vi "Ex 03 - A-Scan + Peaks (Live Update).vi"() -> ()   [LabVIEW 2015]
uses:
  <instrlib>/MicroPulse/Public/Data/Datatypes/MP - data formatting.ctl
  <instrlib>/MicroPulse/Public/Data/Datatypes/MP - amplitude reporting mode.ctl
  <instrlib>/MicroPulse/Public/Data/Datatypes/MP - averaging.ctl
  <instrlib>/MicroPulse/Public/Data/Datatypes/MP - transmit parameters.ctl
  <instrlib>/MicroPulse/Public/Data/Datatypes/MP - pulser voltage.ctl
  <instrlib>/MicroPulse/Public/Data/Datatypes/MP - pulse damping.ctl
  <instrlib>/MicroPulse/Public/Data/Datatypes/MP - test parameters.ctl
  <instrlib>/MicroPulse/Public/Data/Datatypes/MP - receive parameters.ctl
  <instrlib>/MicroPulse/Public/Data/Datatypes/MP - display gate.ctl
  <instrlib>/MicroPulse/Public/Data/Datatypes/MP - waveform type.ctl
  <instrlib>/MicroPulse/Public/Data/Datatypes/MP - analogue filter.ctl
  <instrlib>/MicroPulse/Public/Data/Datatypes/MP - frequency filter.ctl
  <instrlib>/MicroPulse/Public/Data/Datatypes/MP - digital filtering.ctl
  <instrlib>/MicroPulse/Public/Data/Datatypes/MP - high pass filter.ctl
  <instrlib>/MicroPulse/Public/Data/Datatypes/MP - low pass filter.ctl
  <instrlib>/MicroPulse/Public/Data/Datatypes/TCP config.ctl
  <instrlib>/MicroPulse/Public/Data/Datatypes/MP - peak settings.ctl
  <instrlib>/MicroPulse/Public/Data/Datatypes/MP - hysteresis level.ctl
  <instrlib>/MicroPulse/Public/Data/Datatypes/MP - sample frequency.ctl
  <instrlib>/MicroPulse/Public/Data/Datatypes/MP - instrument type.ctl
  <instrlib>/MicroPulse/Public/Data/Datatypes/MP - data output format.ctl
  <instrlib>/MicroPulse/Public/Data/Datatypes/MP - echo gate mode.ctl
  <instrlib>/MicroPulse/MicroPulse_Driver.lvlib
panel:
  in  "PRF":u16=500 caption="[PRF]" min=1 max=20000 step=100 format="%dHz"
  in  "Data Output Format":T1=enum."8-bit Mode"
  out "Instrument Type":T2
  out "Sample Frequency":T3
  out "peak data":cluster{"Time":dbl[], "Level":u16[]}
  in  "Peak Settings":T4={"Upper Threshold"=10, "Hysteresis"=enum."6dB", "# Peaks In Gate"=8} {"# Peaks In Gate" min=1 max=80; "Upper Threshold" min=10}
  in  "Single Scan":bool
  in  "Stop Acquisition":bool
  in  "Start Acquisition":bool
  out "Command List":string
  in  "QUIT":bool
  out "running average PRF":dbl format="%0.2f"
  out "A-Scan + Peaks":cluster{"timebase":dbl[], "data":u16[]}[](graph)
  out "live error out":errorcluster
  out "message count":i32
  out "System Messages":string
  in  "TCP config":T6={"Connection ID"=refnum, "IP address"="10.1.1.2", "host port"=1067, "OC timeout"=5000, "Read timeout"=2000, "Write timeout"=100} {"Write timeout" format="%dms"; "Read timeout" format="%dms"; "OC timeout" format="%dms"}
  in  "Receive Parameters":T7={"Display Gate"={"Start"=0.0, "Length"=100.0}, "Delay"=0.0, "Waveform Type"=enum."Rectified Signal", "Gain"=50.0, "Analogue Filtering"={"Bandpass"=enum."No change", "Smoothing"=1}, "Digital Filtering"={"High Pass Filter"=enum."None", "Low Pass Filter"=enum."None"}} {"Delay" format="%#_g us"; "Display Gate"."Length" min=0.0 max=64000.0 step=1.0 format="%#_g us"; "Display Gate"."Start" min=0.0 max=64000.0 step=1.0 format="%#_g us"; "Analogue Filtering"."Smoothing" min=1 max=11 step=1; "Gain" min=-6.0 max=70.0 step=0.25 format="%.2fdB"}
  in  "Test Parameters":T15={"Test No."=1, "Tx Channel"=1, "Rx Channel"=1} {"Rx Channel" min=1 max=1024; "Tx Channel" min=1 max=1024}
  in  "Transmit Parameters":T16={"Pulse Voltage"=enum."50V", "Pulse Shape"={"Damping"=enum."660W", "Width"=250}} {"Pulse Shape"."Width" min=16 max=1010 step=50 format="%.0fns"}
  in  "Data Formatting":T19={"Amplitude Mode"=enum."Ascan + Peaks", "Averaging"=enum."None", "Coupling Level"=0} {"Coupling Level" max=4095 step=1}
  # "Example 03 - A-scan + Peaks Live Update\n\nSet all controls to the required values\nbefore running the VI.\n\nWhile running, test parameters may be changed."
  # "Channels MUST be set BEFORE running"
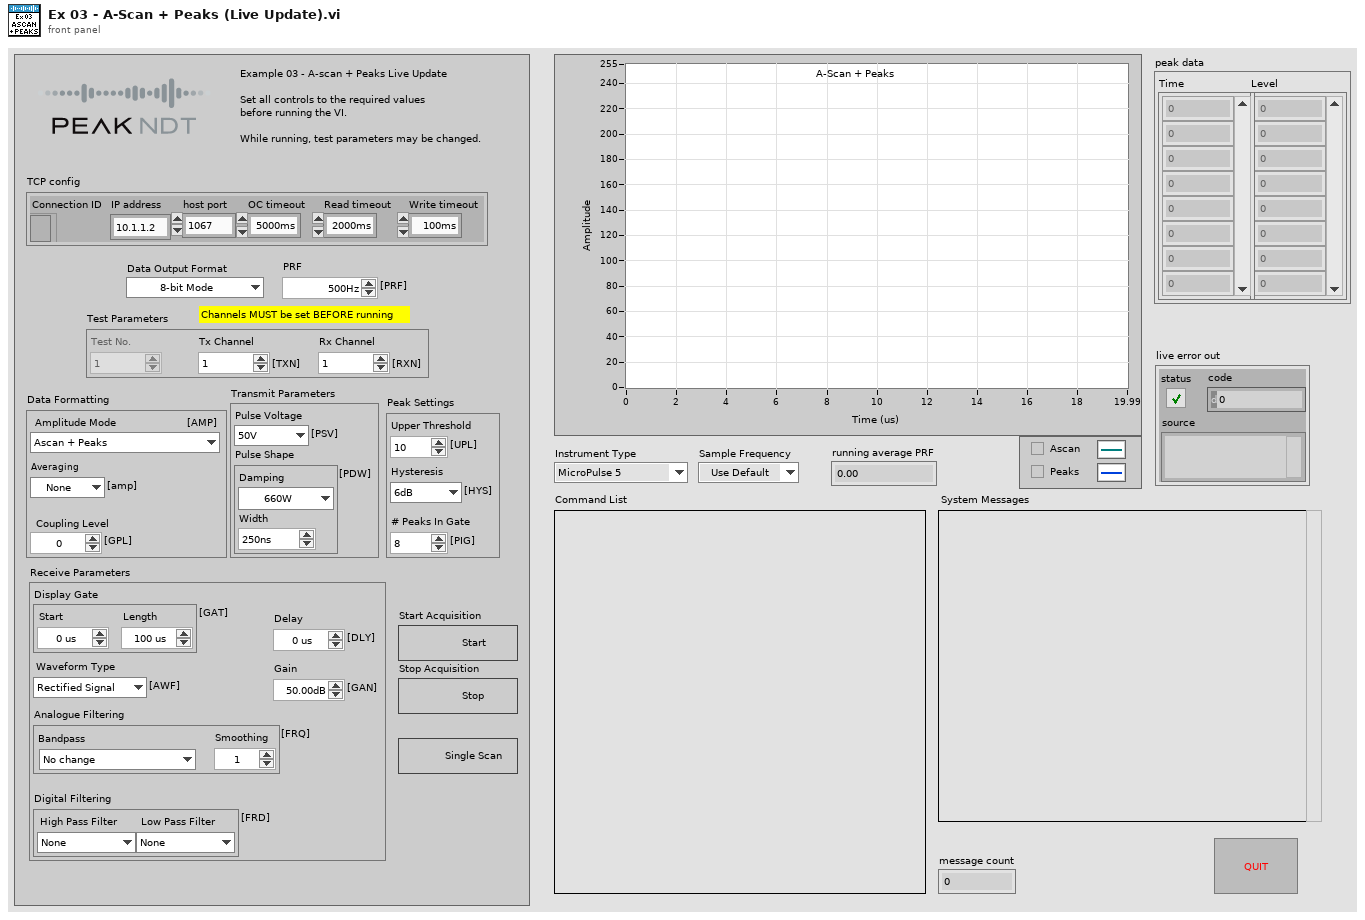
[diagram p1: front panel]
types:
  T1 = typedef "MicroPulse_Driver.lvlib/MP - data output format.ctl" = enum16{"", "8-bit Mode", "10-bit Mode", "12-bit Mode", "16-bit Mode", "8-bit Log Mode", "12-bit Packed Mode"}
  T2 = typedef "MicroPulse_Driver.lvlib/MP - instrument type.ctl" = enum16{"MicroPulse 5", "LT1", "LT2", "LTPA", "MPLT", "MicroPulse 6", "PipeScanner", "<MicroPulse>", "Micropulse 4", "Simulated Data"}
  T3 = typedef "MicroPulse_Driver.lvlib/MP - sample frequency.ctl" = enum16{"Use Default", "200MHz (LT2 only)", "100MHz", "50MHz", "25MHz", "10MHz"}
  T4 = typedef "MicroPulse_Driver.lvlib/MP - peak settings.ctl" = cluster{"Upper Threshold":u16, "Hysteresis":T5, "# Peaks In Gate":u16}
  T5 = typedef "MicroPulse_Driver.lvlib/MP - hysteresis level.ctl" = enum16{"None", "3dB", "6dB", "9dB", "12dB"}
  T6 = typedef "MicroPulse_Driver.lvlib/TCP config.ctl" = cluster{"Connection ID":refnum<k5>, "IP address":string, "host port":u16, "OC timeout":i32, "Read timeout":i32, "Write timeout":i32}
  T7 = typedef "MicroPulse_Driver.lvlib/MP - receive parameters.ctl" = cluster{"Display Gate":T8, "Delay":dbl, "Waveform Type":T9, "Gain":dbl, "Analogue Filtering":T10, "Digital Filtering":T12}
  T8 = typedef "MicroPulse_Driver.lvlib/MP - display gate.ctl" = cluster{"Start":dbl, "Length":dbl}
  T9 = typedef "MicroPulse_Driver.lvlib/MP - waveform type.ctl" = enum16{"Rectified Signal", "RF Signal", "+Half Wave", "-Half Wave"}
  T10 = typedef "MicroPulse_Driver.lvlib/MP - analogue filter.ctl" = cluster{"Bandpass":T11, "Smoothing":u16}
  T11 = typedef "MicroPulse_Driver.lvlib/MP - frequency filter.ctl" = enum16{"No change", "1MHz Bandpass", "2MHz Bandpass", "4MHz Bandpass", "5MHz Bandpass", "10MHz Bandpass", "2.5-18MHz Broadband", "0.75-12MHz  Broadband", "0.5MHz Bandpass", "5MHz 2nd Order TOFD", "10MHz 2nd Order TOFD", "3.0-25MHz Broadband", "3.0-30MHz Broadband"}
  T12 = typedef "MicroPulse_Driver.lvlib/MP - digital filtering.ctl" = cluster{"High Pass Filter":T13, "Low Pass Filter":T14}
  T13 = typedef "MicroPulse_Driver.lvlib/MP - high pass filter.ctl" = enum16{"None", "0.7MHz", "1.5MHz", "4.0MHz", "7.5MHz", "10.0MHz", "User Defined"}
  T14 = typedef "MicroPulse_Driver.lvlib/MP - low pass filter.ctl" = enum16{"None", "1.8MHz", "3.0MHz", "6.0MHz", "8.0MHz", "12.0MHz", "User Defined"}
  T15 = typedef "MicroPulse_Driver.lvlib/MP - test parameters.ctl" = cluster{"Test No.":u32, "Tx Channel":u32, "Rx Channel":u32}
  T16 = typedef "MicroPulse_Driver.lvlib/MP - transmit parameters.ctl" = cluster{"Pulse Voltage":T17, "Pulse Shape":cluster{"Damping":T18, "Width":u32}}
  T17 = typedef "MicroPulse_Driver.lvlib/MP - pulser voltage.ctl" = enum16{"50V", "100V", "150V", "200V", "250V", "300V"}
  T18 = typedef "MicroPulse_Driver.lvlib/MP - pulse damping.ctl" = enum16{"660W", "458W", "220W", "149W", "102W", "82W", "63W", "51W"}
  T19 = typedef "MicroPulse_Driver.lvlib/MP - data formatting.ctl" = cluster{"Amplitude Mode":T20, "Averaging":T21, "Coupling Level":u32}
  T20 = typedef "MicroPulse_Driver.lvlib/MP - amplitude reporting mode.ctl" = enum16{"1st Peak in gate", "Maximum Peak in gate", "All Peaks", "Ascan Data", "1st Threshold Crossing Peak", "Ascan + Peaks", "All Peaks for Multigate", "Peaks + Ascan for Multigate", "Peaks + P_Ascan for Multigate", "Full Matrix Capture"}
  T21 = typedef "MicroPulse_Driver.lvlib/MP - averaging.ctl" = enum16{"None", "2", "4", "8", "16", "32", "64", "128", "256"}
  T22 = typedef "MicroPulse_Driver.lvlib/MP - echo gate mode.ctl" = enum16{"Echo Trigger OFF", "Echo Gate Display Mode", "Echo Trigger ON", "Multi Gate or FMC Mode", "Reserved", "PA - Echo Trigger ON"}
  T23 = typedef "MicroPulse_Driver.lvlib/MP-Registry Data-Cluster.ctl" = cluster{"Instrument Type":T2, "Serial #":u64, "Sample Frequency":T3, "dt (us)":dbl, "DOF":T1, "Material Velocity":dbl, "Asynch Reads":T24, "NUM of Tests":u32, "System Details":T25, "Gates":T27[], "Encoders":T31[], "CMD LUT":variant, "Command List":string}
  T24 = typedef "MicroPulse_Driver.lvlib/MP - asynch read mode.ctl" = enum16{"Disabled", "Enabled"}
  T25 = typedef "MicroPulse_Driver.lvlib/MP - general system status.ctl" = cluster{"System Type":T2, "Serial No.":u64, "Channels":cluster{"Conv":u8, "PA":u16, "Extra":u32}, "Sample Frequency":cluster{"Default":u8, "Actual":u8}, "Software Versions":string, "Data Output Format":cluster{"Default":T1, "Actual":T1}, "Temperatures":cluster{"System":u8, "Processor":u8, "Slave Sys":u8, "Slave Proc":u8}, "Tx Buffer Size":u32, "System Error":string, "No. of Cards":u8, "DAC Gain":i16, "Uptimes":cluster{"since Power":u32, "since RSTS":u32, "since SRST":u32}, "Voltages":cluster{"Nominal":dbl, "Measured":dbl, "Difference":dbl}[], "Interface Cards":T26[]}
  T26 = typedef "MicroPulse_Driver.lvlib/MP - interface card status.ctl" = cluster{"Status":u8, "Map":u8, "Board - T":u8, "FPGA - T":u8, "PAIF Status":string, "Version":string}
  T27 = typedef "MicroPulse_Driver.lvlib/MP - Registry Gates.ctl" = cluster{"Display Gate":T8, "ETM Mode":T22, "Echo Gate":T28, "Insp Gates":T29[]}
  T28 = typedef "MicroPulse_Driver.lvlib/MP - echo gate parameters.ctl" = cluster{"Start (us)":dbl, "Length (us)":dbl, "Threshold":u16, "Colour":u32}
  T29 = typedef "MicroPulse_Driver.lvlib/MP - multigate inspection gate parameters.ctl" = cluster{"Start (us)":dbl, "Length (us)":dbl, "Threshold":u16, "Enabled?":bool, "Max # Peaks":u16, "Hysteresis":T5, "Mode":T30, "Inverted?":bool, "Colour ":u32}
  T30 = typedef "MicroPulse_Driver.lvlib/MP - multigate mode.ctl" = enum16{"1st Peak in Gate", "Largest Peak In Gate", "All Peaks In Gate", "1st Threshold Crossing"}
  T31 = typedef "MicroPulse_Driver.lvlib/MP - encoder settings.ctl" = cluster{"Encoder Type":T32, "Counts/mm":u32, "Enable Termination?":bool, "Multiplier":u32, "Backlash Period (s)":dbl, "Encoder Filter":u32}
  T32 = typedef "MicroPulse_Driver.lvlib/MP - encoder type.ctl" = enum16{"Quadrature", "Step/Direction"}
  T33 = typedef "MicroPulse_Driver.lvlib/MP - scan data info.ctl" = cluster{"Message Header":u16, "Error Message":u16, "Test No.":u32, "Channel No.":u8, "Sweep No.":u32, "Gate No.":u32, "DOF":T1, "retain data":T34, "scan data":u16[], "scan length":i32, "scan index":i32, "peak data":cluster{"timebase":u16[], "data":u16[]}, "#peaks":i32, "PRF":dbl, "IP":cluster{"Axis No.":u8, "Location":u32, "MIP location":u32, "MIP?":bool}, "echo range":u16, "ETG":bool, "CAL 0 complete":bool, "Axis Positions":T35}
  T34 = typedef "MicroPulse_Driver.lvlib/MP - retain scan.ctl" = enum16{"None", "Ascan", "Peaks"}
  T35 = typedef "MicroPulse_Driver.lvlib/MP - axis positions (LLC).ctl" = cluster{"Axis 1":u32, "Axis 2":u32, "Axis 3":u32, "Axis 4":u32, "Status":u8}
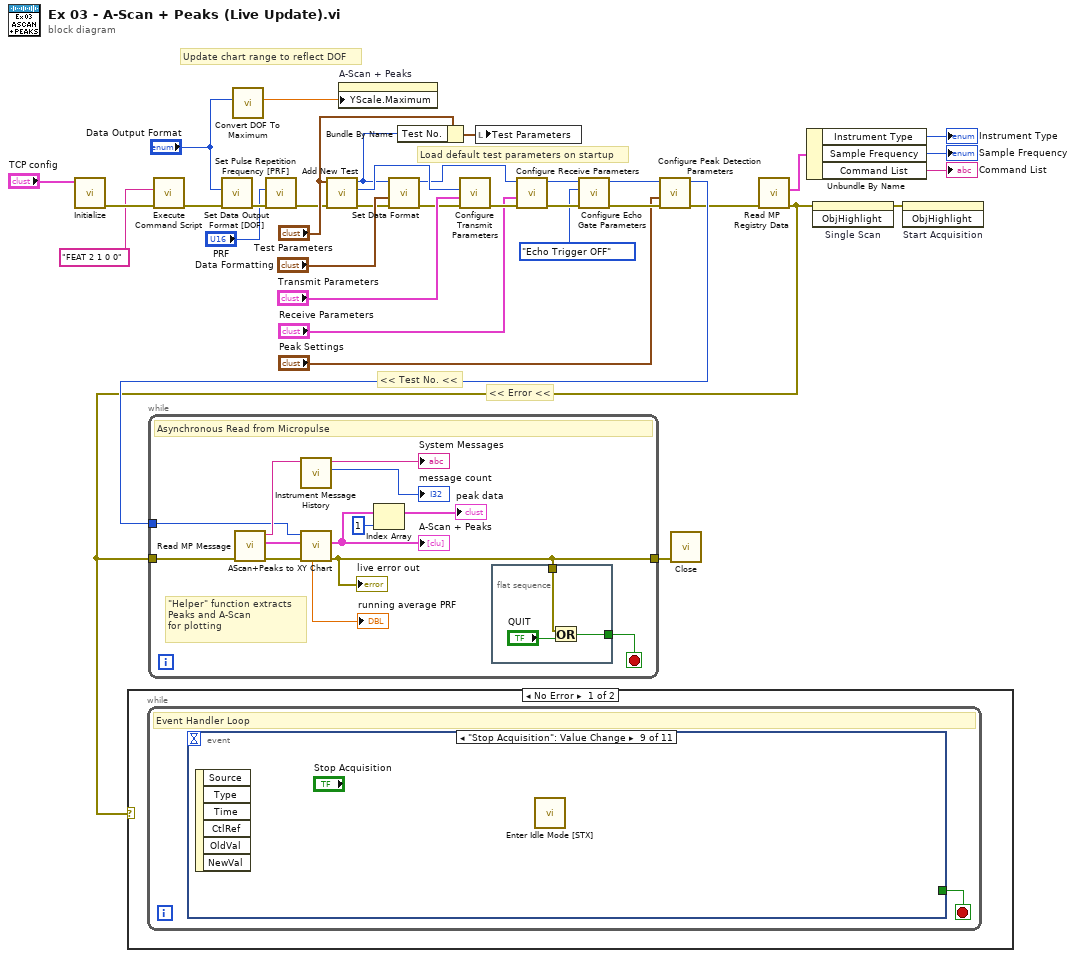
[diagram p0: block diagram]
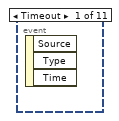
[diagram p2: hidden frame]
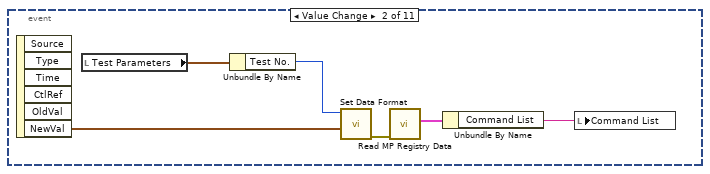
[diagram p3: hidden frame]
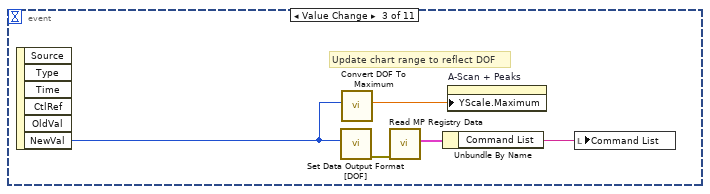
[diagram p4: hidden frame]
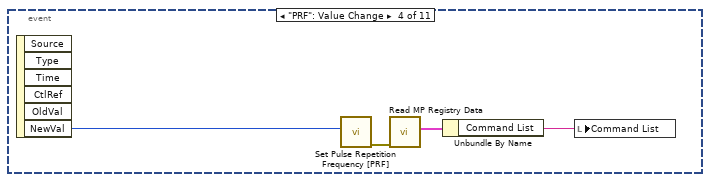
[diagram p5: hidden frame]
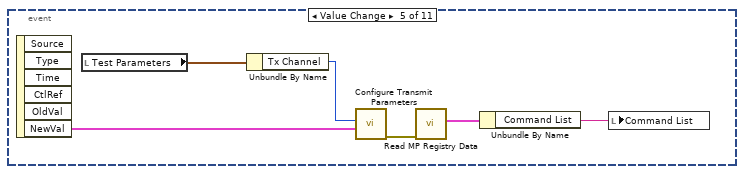
[diagram p6: hidden frame]
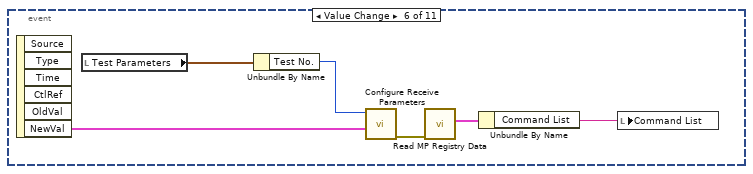
[diagram p7: hidden frame]
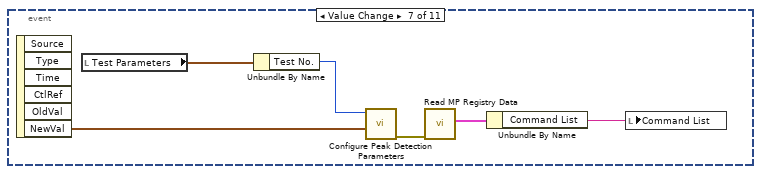
[diagram p8: hidden frame]
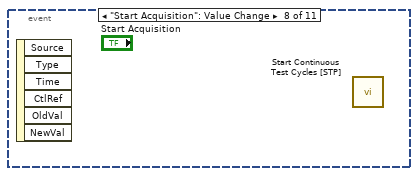
[diagram p9: hidden frame]
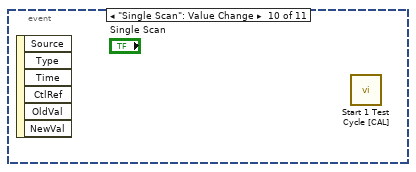
[diagram p10: hidden frame]
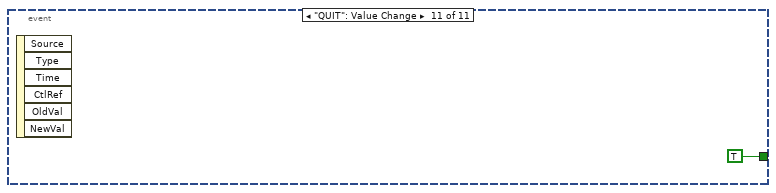
[diagram p11: hidden frame]
diagram:
  # "Update chart range to reflect DOF"
  # "<< Error <<"
  # "<< Test No. <<"
  # "Load default test parameters on startup"
  n1 = call <instrlib>:"Initialize.vi"("TCP config"="TCP config") -> ("error out"=w2:errorcluster)  [unwired: 9 in, 1 out]
  n2 = call <instrlib>:"Execute Command Script.vi"("error in (no error)"=w2, "String in"="FEAT 2 1 0 0") -> ("error out"=w3:errorcluster)  [unwired: 7 in, 2 out]
  n3 = call <instrlib>:"Set Data Output Format [DOF].vi"("error in (no error)"=w3, "Mode"="Data Output Format") -> ("error out"=w8:errorcluster)  [unwired: 8 in, 1 out]
  n4 = call <instrlib>:"Convert DOF To Maximum.vi"("Data Output Format"="Data Output Format") -> ("Data Maximum"=w5:dbl)  [unwired: 10 in]
  n5 = call <instrlib>:"Set Pulse Repetition Frequency [PRF].vi"("error in (no error)"=w8, "Frequency (Hz)"="PRF") -> ("error out"=w7:errorcluster)  [unwired: 8 in, 1 out]
  n6 = call <instrlib>:"Add New Test.vi"("error in (no error)"=w7, "Test Parameters"="Test Parameters") -> ("error out"=w26:errorcluster, "Tx Channel out"=w25:u32, "Test No. out"=w10:u32)  [unwired: 6 in, 1 out]
  n7 = property on="A-Scan + Peaks" class="XYGraph (strict)"("YScale.Maximum"=w5) -> ()  [unwired: 2 in, 2 out]
  n8 = call <instrlib>:"Set Data Format.vi"("error in (no error)"=w26, "Data Formatting"="Data Formatting", "Test No."=w10) -> ("error out"=w31:errorcluster, "Test No. out"=w24:u32)  [unwired: 6 in, 1 out]
  n9 = Bundle By Name(cluster="Test Parameters", "Test No."=w10) -> (w9:T15)
  n10 = call <instrlib>:"Configure Transmit Parameters.vi"("error in (no error)"=w31, "Transmit Parameters"="Transmit Parameters", "Tx Channel"=w25) -> ("error out"=w32:errorcluster)  [unwired: 7 in, 1 out]
  n11 = local write "Test Parameters"(w9) -> ()
  n12 = call <instrlib>:"Configure Receive Parameters.vi"("error in (no error)"=w32, "Receive Parameters"="Receive Parameters", "Test No."=w24) -> ("error out"=w30:errorcluster, "Test No. out"=w23:u32)  [unwired: 6 in, 1 out]
  n13 = call <instrlib>:"Configure Echo Gate Parameters.vi"("error in (no error)"=w30, "Echo Trigger Mode"=MP_-_echo_gate_mode."Echo Trigger OFF" ("ETM Mode"), "Test Number"=w23) -> ("error out"=w20:errorcluster, "Test Number Out"=w22:u32)  [unwired: 6 in, 1 out]
  n14 = call <instrlib>:"Configure Peak Detection Parameters.vi"("error in (no error)"=w20, "Peak Settings"="Peak Settings", "Test Number"=w22) -> ("error out"=w19:errorcluster, "Test Number Out"=w21:u32)  [unwired: 6 in, 1 out]
  n15 = call <instrlib>:"Read MP Registry Data.vi"("error in (no error)"=w19) -> ("error out"=w15:errorcluster, "Micropulse Data"=w17:T23)  [unwired: 7 in, 2 out]
  n16 = case shown="No Error" w15 {
    frame No Error {
      n17 = while {
        stop <- w36 stop-if-true
        # "Event Handler Loop"
        n18 = event shown="[8] \"Stop Acquisition\": Value Change" {
          selector: _ -> [_ _ _ _ _ _ _ _ _ _ _]
          dyn-events: _ -> [_ _ _ _ _ _ _ _ _ _ _]
          timeout: _ -> [_ _ _ _ _ _ _ _ _ _ _]
          tunnel: [_ _ _ _ _ _ _ _ _ _ TRUE ("stop")] -> w36
          event Timeout {
            n19 = event-data() -> ()  [unwired: 1 in, 3 out]
          }
          event Value Change {
            n20 = event-data() -> ("NewVal"=w42:T19)  [unwired: 1 in, 5 out]
            n21 = local read "Test Parameters"() -> (w41:T15)
            n22 = Unbundle By Name(w41) -> ("Test No."=w40:u32)
            n23 = call <instrlib>:"Set Data Format.vi"("Data Formatting"=w42, "Test No."=w40) -> ("error out"=w38:errorcluster)  [unwired: 7 in, 2 out]
            n24 = call <instrlib>:"Read MP Registry Data.vi"("error in (no error)"=w38) -> ("Micropulse Data"=w39:T23)  [unwired: 7 in, 3 out]
            n25 = Unbundle By Name(w39) -> ("Command List"=w37:string)
            n26 = local write "Command List"(w37) -> ()
          }
          event Value Change {
            # "Update chart range to reflect DOF"
            n27 = event-data() -> ("NewVal"=w43:T1)  [unwired: 1 in, 5 out]
            n28 = call <instrlib>:"Set Data Output Format [DOF].vi"("Mode"=w43) -> ("error out"=w46:errorcluster)  [unwired: 9 in, 1 out]
            n29 = call <instrlib>:"Convert DOF To Maximum.vi"("Data Output Format"=w43) -> ("Data Maximum"=w44:dbl)  [unwired: 10 in]
            n30 = call <instrlib>:"Read MP Registry Data.vi"("error in (no error)"=w46) -> ("Micropulse Data"=w47:T23)  [unwired: 7 in, 3 out]
            n31 = Unbundle By Name(w47) -> ("Command List"=w45:string)
            n32 = property on="A-Scan + Peaks" class="XYGraph (strict)"("YScale.Maximum"=w44) -> ()  [unwired: 2 in, 2 out]
            n33 = local write "Command List"(w45) -> ()
          }
          event "PRF": Value Change {
            n34 = event-data() -> ("NewVal"=w48:u16)  [unwired: 1 in, 5 out]
            n35 = call <instrlib>:"Set Pulse Repetition Frequency [PRF].vi"("Frequency (Hz)"=w48) -> ("error out"=w50:errorcluster)  [unwired: 9 in, 1 out]
            n36 = call <instrlib>:"Read MP Registry Data.vi"("error in (no error)"=w50) -> ("Micropulse Data"=w51:T23)  [unwired: 7 in, 3 out]
            n37 = Unbundle By Name(w51) -> ("Command List"=w49:string)
            n38 = local write "Command List"(w49) -> ()
          }
          event Value Change {
            n39 = event-data() -> ("NewVal"=w56:T16)  [unwired: 1 in, 5 out]
            n40 = local read "Test Parameters"() -> (w57:T15)
            n41 = Unbundle By Name(w57) -> ("Tx Channel"=w55:u32)
            n42 = call <instrlib>:"Configure Transmit Parameters.vi"("Transmit Parameters"=w56, "Tx Channel"=w55) -> ("error out"=w53:errorcluster)  [unwired: 8 in, 1 out]
            n43 = call <instrlib>:"Read MP Registry Data.vi"("error in (no error)"=w53) -> ("Micropulse Data"=w54:T23)  [unwired: 7 in, 3 out]
            n44 = Unbundle By Name(w54) -> ("Command List"=w52:string)
            n45 = local write "Command List"(w52) -> ()
          }
          event Value Change {
            n46 = event-data() -> ("NewVal"=w59:T7)  [unwired: 1 in, 5 out]
            n47 = local read "Test Parameters"() -> (w63:T15)
            n48 = Unbundle By Name(w63) -> ("Test No."=w62:u32)
            n49 = call <instrlib>:"Configure Receive Parameters.vi"("Receive Parameters"=w59, "Test No."=w62) -> ("error out"=w61:errorcluster)  [unwired: 7 in, 2 out]
            n50 = call <instrlib>:"Read MP Registry Data.vi"("error in (no error)"=w61) -> ("Micropulse Data"=w60:T23)  [unwired: 7 in, 3 out]
            n51 = Unbundle By Name(w60) -> ("Command List"=w58:string)
            n52 = local write "Command List"(w58) -> ()
          }
          event Value Change {
            n53 = event-data() -> ("NewVal"=w65:T4)  [unwired: 1 in, 5 out]
            n54 = local read "Test Parameters"() -> (w69:T15)
            n55 = Unbundle By Name(w69) -> ("Test No."=w68:u32)
            n56 = call <instrlib>:"Configure Peak Detection Parameters.vi"("Peak Settings"=w65, "Test Number"=w68) -> ("error out"=w67:errorcluster)  [unwired: 7 in, 2 out]
            n57 = call <instrlib>:"Read MP Registry Data.vi"("error in (no error)"=w67) -> ("Micropulse Data"=w66:T23)  [unwired: 7 in, 3 out]
            n58 = Unbundle By Name(w66) -> ("Command List"=w64:string)
            n59 = local write "Command List"(w64) -> ()
          }
          event "Start Acquisition": Value Change {
            n60 = event-data() -> ()  [unwired: 1 in, 6 out]
            n61 = call <instrlib>:"Start Continuous Test Cycles [STP].vi"() -> ()  [unwired: 10 in, 2 out]
          }
          event "Stop Acquisition": Value Change {
            n62 = event-data() -> ()  [unwired: 1 in, 6 out]
            n63 = call <instrlib>:"Enter Idle Mode [STX].vi"() -> ()  [unwired: 10 in, 2 out]
          }
          event "Single Scan": Value Change {
            n64 = event-data() -> ()  [unwired: 1 in, 6 out]
            n65 = call <instrlib>:"Start 1 Test Cycle [CAL].vi"() -> ()  [unwired: 10 in, 2 out]
          }
          event "QUIT": Value Change {
            n66 = event-data() -> ()  [unwired: 1 in, 6 out]
          }
        }
      }
    }
    frame Error {
    }
  }
  n67 = while {
    tunnel: [w72] -> w29
    tunnel: w15 -> [w79]
    tunnel: w21 -> [w77]
    stop <- w82 stop-if-true
    # "\"Helper\" function extracts\nPeaks and A-Scan\nfor plotting"
    # "Asynchronous Read from Micropulse"
    n68 = call <instrlib>:"Read MP Message.vi"("error in (no error)"=w79) -> ("error out"=w78:errorcluster, "scan data info"=w76:T33, "Instrument Message"=w81:string)  [unwired: 6 in, 2 out]
    n69 = call <instrlib>:"Instrument Message History.vi"("Instrument Message"=w81) -> ("Message Count"=→"message count":i32, "Message History out"=→"System Messages":string)  [unwired: 9 in]
    n70 = call <instrlib>:"AScan+Peaks to XY Chart.vi"("error in (no error)"=w78, "scan data info"=w76, "Test No."=w77) -> ("error out"=w72:errorcluster, "AScan+Peaks"=w75:cluster{"timebase":dbl[], "data":u16[]}[], "Running Average PRF"=→"running average PRF":dbl)  [unwired: 3 in, 3 out]
    "A-Scan + Peaks" <- w75
    "live error out" <- w72
    n71 = Index Array(array=w75, index=1) -> (element=→"peak data":cluster{"timebase":dbl[], "data":u16[]})
    n72 = flat-sequence {
      tunnel: [w85] -> w82
      tunnel: w72 -> [w84]
      frame #0 {
        n73 = Or(x=w84, y="QUIT") -> (x .or. y?=w85:bool)
      }
    }
  }
  n74 = call <instrlib>:"Close.vi"("error in (no error)"=w29) -> ()  [unwired: 9 in, 2 out]
  n75 = Unbundle By Name(w17) -> ("Instrument Type"=→"Instrument Type":T2, "Sample Frequency"=→"Sample Frequency":T3, "Command List"=→"Command List":string)
  n76 = invoke on="Single Scan" class="Bool" method="ObjHighlight"(error in=w15) -> (error out=w14:errorcluster)  [unwired: 2 in, 2 out]
  n77 = invoke on="Start Acquisition" class="Bool" method="ObjHighlight"(error in=w14) -> ()  [unwired: 2 in, 3 out]
